vi "PlaySingle.vi"(0 "Program Interface in":refnum<class "Program Interface.lvclass">, 1 "robot":refnum<class "Universal Robot.lvclass">, 5 "error in (no error)":errorcluster, 9 "Subpanel":refnum<vi>) -> (14 "Program Interface out":refnum<class "Program Interface.lvclass">, 15 "programReturnStatus":T1=enum."Complete", 19 "error out":errorcluster)   [LabVIEW 2019, in "Program Interface.lvclass"]
uses:
  Program Interface.lvclass
  Robot/Universal Robot/Universal Robot.lvclass
  Robot/Universal Robot/ProgramReturnStatus.ctl
  Program Interface.lvclass/Program Interface.ctl
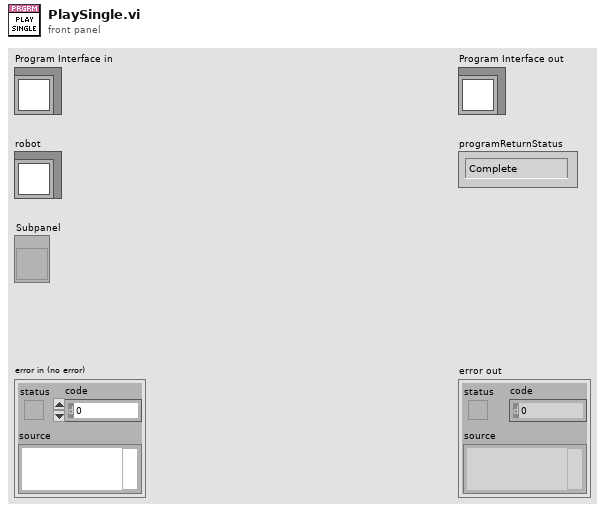
[diagram p1: front panel]
types:
  T1 = typedef "Universal Robot.lvclass/ProgramReturnStatus.ctl" = enum16{"Incomplete", "Complete", "Stopped", "Error", "Faulted", "Timeout"}
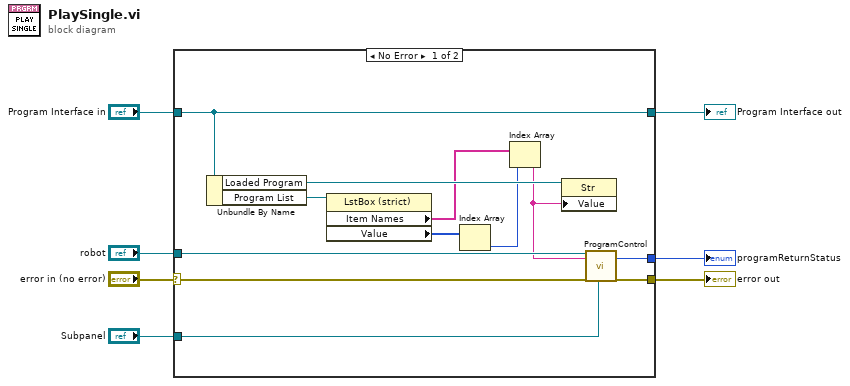
[diagram p0: block diagram]
diagram:
  n1 = case shown="No Error" "error in (no error)" {
    selector: "error in (no error)" -> [w18 w21]
    tunnel: [w17 w21] -> w6
    tunnel: [w19 w20] -> w4
    tunnel: "Program Interface in" -> [w19 w20]
    tunnel: "robot" -> [w15 _]
    tunnel: [w13 _] -> w2
    tunnel: "Subpanel" -> [w12 _]
    frame No Error {
      n2 = Unbundle By Name(w19) -> ("Loaded Program"=w14:refnum<vi>, "Program List"=w16:refnum<vi>)
      n3 = property class="LstBox (strict)"(reference=w16) -> ("Item Names"=w11:string[], "Value"=w10:i32[])  [unwired: 1 in, 2 out]
      n4 = Index Array(array=w10) -> (element=w9:i32)  [unwired: 1 in]
      n5 = Index Array(array=w11, index=w9) -> (element=w8:string)
      n6 = property class="Str"(reference=w14, "Value"=w8) -> ()  [unwired: 1 in, 2 out]
      n7 = call-dynamic "ProgramControl.vi"("Universal Robot.lvclass in"=w15, "Program"=w8, "error in (no error)"=w18, "Subpanel"=w12) -> ("programReturnStatus"=w13:T1, "error out"=w17:errorcluster)  [unwired: 13 in, 1 out]
    }
    frame Error {
    }
  }
  "error out" <- w6
  "Program Interface out" <- w4
  "programReturnStatus" <- w2
